vi "Stop Core.vi"(10 "final error code":i32, 11 "UserManagement in":refnum<class "UserManagement.lvclass">) -> (3 "UserManagement out":refnum<class "UserManagement.lvclass">)   [LabVIEW 2019, in "UserManagement.lvlib" / "UserManagement.lvclass"]
uses:
  UserManagement.lvclass
  UserManagement.lvclass/UserManagement.ctl
  <vilib>/NI/Event Source Actor/Event Source/Event Source/Event Source.lvclass
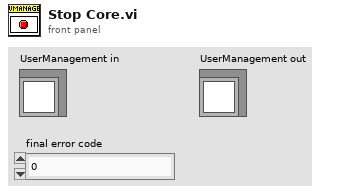
[diagram p1: front panel]
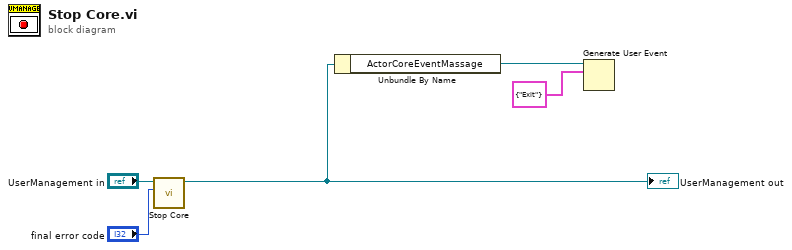
[diagram p0: block diagram]
diagram:
  n1 = call-parent "Stop Core.vi"("final error code"="final error code", "Event Source In"="UserManagement in") -> ("Event Source Out"=w3:refnum<class "UserManagement.lvclass">)  [unwired: 9 in]
  "UserManagement out" <- w3
  n2 = Unbundle By Name(w3) -> ("ActorCoreEventMassage"=w2:refnum<user-event>)
  n3 = Generate User Event(user event=w2, event data cluster=cluster{"ActorCoreEventMassage":string} {"ActorCoreEventMassage"="Exit"} ("event data")) -> ()  [unwired: 2 in, 2 out]
